vi "ConfigDelayScreen.vi"() -> ()   [LabVIEW 2011]
panel:
  out "x+1":i32 format="%d %"
  out "Bar":u8(slide) scale=0.0..100.0
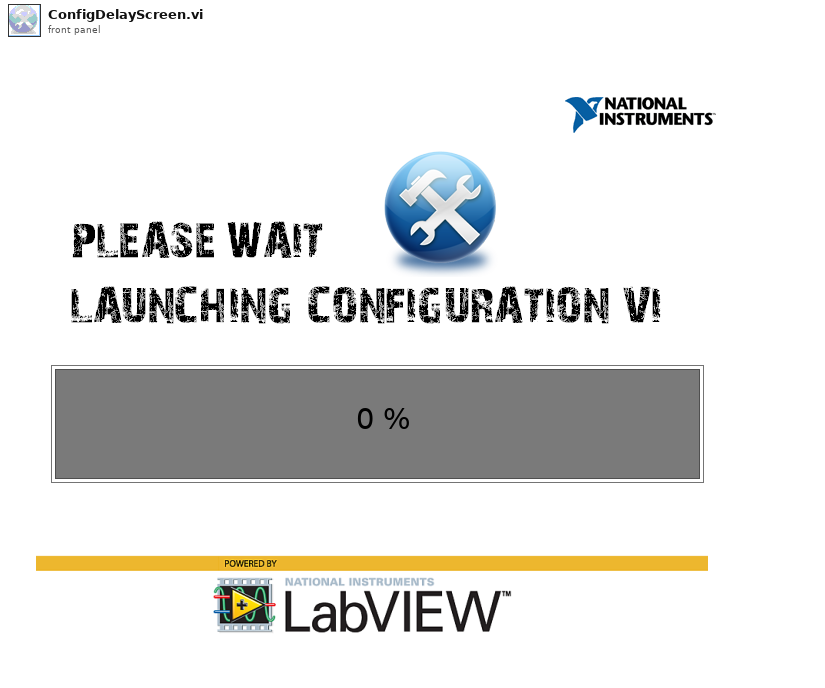
[diagram p1: front panel]
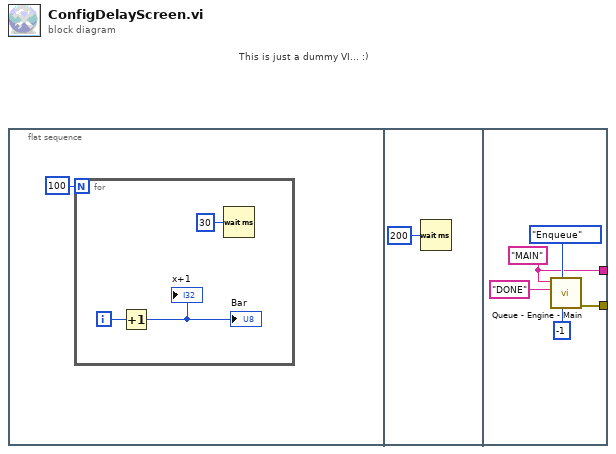
[diagram p0: block diagram]
diagram:
  # "This is just a dummy VI... :)"
  n1 = flat-sequence {
    tunnel: [w7] -> _
    tunnel: [w6] -> _
    frame #0 {
      n2 = for {
        N: 100 -> [_]
        i -> [w4]
        n3 = Increment(x=w4) -> (x+1=→"Bar" →"x+1":i32)
        n4 = Wait (ms)(milliseconds to wait=u32 30) -> ()  [unwired: 1 out]
      }
    }
    frame #1 {
      n5 = Wait (ms)(milliseconds to wait=u32 200) -> ()  [unwired: 1 out]
    }
    frame #2 {
      w6 = "MAIN" ("Queue Name In")
      n6 = call "Queue - Engine - Main.vi"("timeout in ms (-1)"=-1, "Operation"=enum16{"Enqueue", "Dequeue", "Flush", "Release"}."Enqueue", "Queue Data In"="DONE" ("Queue Name In"), "Queue Name In"=w6) -> ("error out"=w7:errorcluster)  [unwired: 5 in, 2 out]
    }
  }
